vi "Assy_POKAYOKE_03_41_00_PM.vi"() -> ()   [LabVIEW 2020]
panel:
  in  "Assy_POKAYOKE":T1
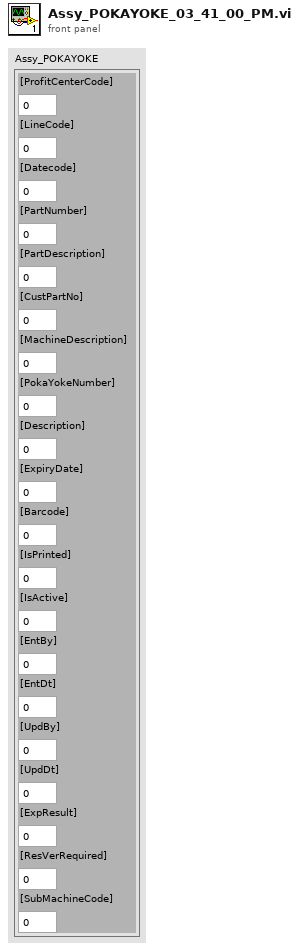
[diagram p1: front panel]
types:
  T1 = cluster{"[ProfitCenterCode]":dbl, "[LineCode]":dbl, "[Datecode]":dbl, "[PartNumber]":dbl, "[PartDescription]":dbl, "[CustPartNo]":dbl, "[MachineDescription]":dbl, "[PokaYokeNumber]":dbl, "[Description]":dbl, "[ExpiryDate]":dbl, "[Barcode]":dbl, "[IsPrinted]":dbl, "[IsActive]":dbl, "[EntBy]":dbl, "[EntDt]":dbl, "[UpdBy]":dbl, "[UpdDt]":dbl, "[ExpResult]":dbl, "[ResVerRequired]":dbl, "[SubMachineCode]":dbl}
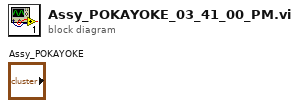
[diagram p0: block diagram]
diagram:
